vi "CO MFR sw 3.vi"(8 "Increment":dbl, 9 "Bottle conc":dbl, 10 "C_CO":dbl, 11 "Flow rate":dbl) -> (3 "CO MFR":dbl)   [LabVIEW 2014]
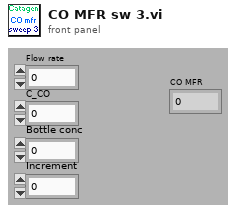
[diagram p1: front panel]
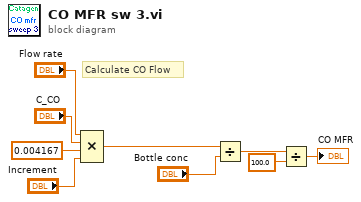
[diagram p0: block diagram]
diagram:
  # "Calculate CO Flow"
  n1 = Compound Arithmetic op=MULTIPLY("Flow rate", "C_CO", 0.004167 ("x"), "Increment") -> (w5:dbl)
  n2 = Divide(x=w5, y="Bottle conc") -> (x/y=w4:dbl)
  n3 = Divide(x=w4, y=100.0) -> (x/y=→"CO MFR":dbl)
